vi "Dispatch Message.vi"(8 "error in (no error)":errorcluster, 10 "TcpPayload":T1, 11 "Remote Messaging Module in":refnum<class "Remote Messaging Module.lvclass">) -> (0 "error out":errorcluster, 3 "Remote Messaging Module out":refnum<class "Remote Messaging Module.lvclass">)   [LabVIEW 2020, in "Volatus.lvlib" / "Remote Messaging Module.lvclass"]
uses:
  Remote Messaging Module.lvclass
  C:/dev/lv20CE/relink/lv-volatus/Volatus/Module/Module.lvclass
  lv-vecto/Vecto/proto/TcpPayload/Data.ctl
  Module/Module.lvclass/Module.ctl
  Module Identity/Module Identity.lvclass/Module Identity.ctl
  MessageQ/MessageQ.lvclass/MessageQ.ctl
  Event Level.ctl
  Remote Messaging Module.lvclass/Remote Messaging Module.ctl
  Module Identity/Module Identity.lvclass
  C:/dev/lv20CE/relink/lv-volatus/Volatus/Identity/Identity.lvclass
  Module/Module.lvclass
  MessageQ/MessageQ.lvclass
  VolatusAPI/VolatusAPI.lvclass
  Volatus.lvlib
  lv-vecto/Vecto/proto/TcpPayload/TcpPayload.lvlib
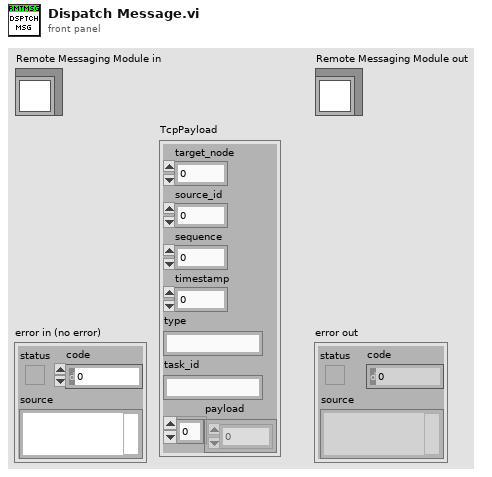
[diagram p1: front panel]
types:
  T1 = typedef "TcpPayload.lvlib/Data.ctl" = cluster{"target_node":u32, "source_id":u32, "sequence":u32, "timestamp":i64, "type":string, "task_id":string, "payload":u8[]}
  T2 = typedef "Volatus.lvlib/Event Level.ctl" = enum16{"Debug", "Info", "Warning", "Error"}
  T3 = typedef "Volatus.lvlib/Remote Messaging Module.lvclass/Type Handler.ctl" = cluster{"Msg ID":string, "MsgQ":refnum<class "MessageQ.lvclass">}
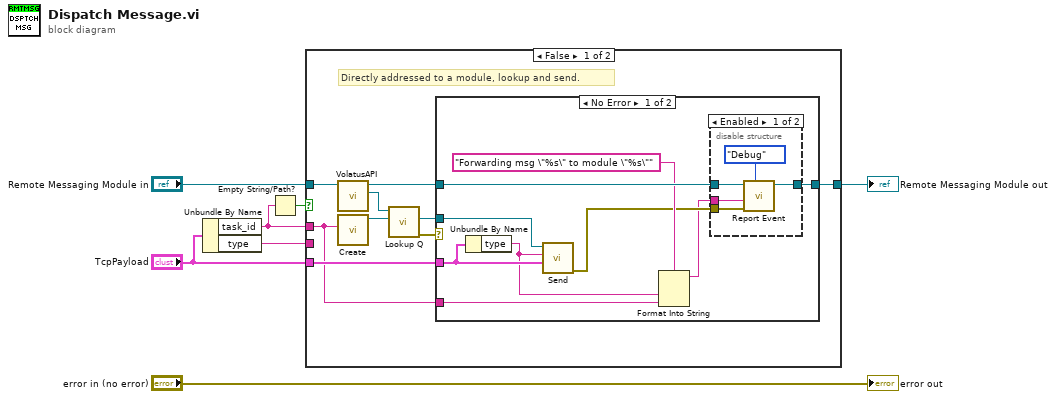
[diagram p0: block diagram]
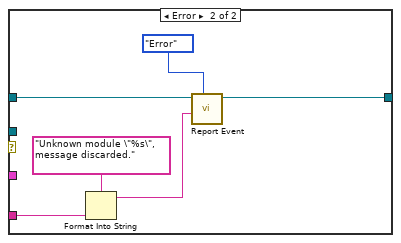
[diagram p3: hidden frame]
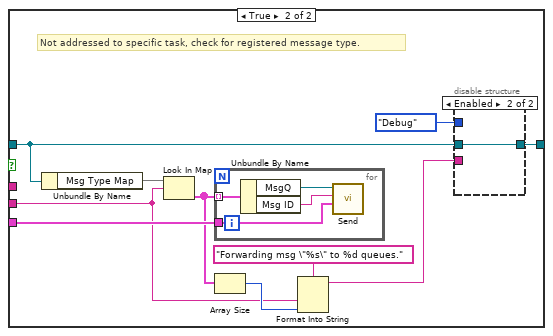
[diagram p4: hidden frame]
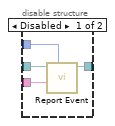
[diagram p5: hidden frame]
diagram:
  n1 = Unbundle By Name("TcpPayload") -> ("task_id"=w2:string, "type"=w4:string)
  n2 = Empty String/Path?(string/path=w2) -> (empty?=w5:bool)
  n3 = case shown="False" w5 {
    tunnel: "Remote Messaging Module in" -> [w16 w45]
    tunnel: w4 -> [_ w41]
    tunnel: "TcpPayload" -> [w11 w46]
    tunnel: w2 -> [w9 _]
    tunnel: [w8 w40] -> w1
    frame False {
      # "Directly addressed to a module, lookup and send."
      n4 = call "VolatusAPI.vi"("Module in"=w16) -> ("VolatusAPI"=w15:refnum<class "VolatusAPI.lvclass">, "Module out"=w10:refnum<class "Remote Messaging Module.lvclass">)  [unwired: 9 in]
      n5 = call "Create.vi"("ID"=w9) -> ("Module Identity out"=w14:refnum<class "Module Identity.lvclass">)  [unwired: 10 in]
      n6 = call "Lookup Q.vi"("Identity"=w14, "VolatusAPI in"=w15) -> ("error out"=w13:errorcluster, "MessageQ"=w12:refnum<class "MessageQ.lvclass">)  [unwired: 7 in, 1 out]
      n7 = case shown="No Error" w13 {
        tunnel: w12 -> [w25 _]
        tunnel: w11 -> [w24 _]
        tunnel: w10 -> [w23 w37]
        tunnel: w9 -> [w20 w34]
        tunnel: [w17 w32] -> w8
        frame No Error {
          n8 = Unbundle By Name(w24) -> ("type"=w21:string)
          n9 = call "Send.vi"("Data"=w24, "ID"=w21, "MessageQ in"=w25) -> ("error out"=w19:errorcluster)  [unwired: 7 in, 1 out]
          n10 = Format Into String(format string="Forwarding msg \"%s\" to module \"%s\"", w21, w20) -> (resulting string=w18:string)  [unwired: 2 in, 1 out]
          n11 = disable-structure shown="Enabled" {
            disable-tunnel: w23 -> [w30 w31]
            disable-tunnel: w19 -> [w29 _]
            disable-tunnel: w18 -> [w28 _]
            disable-tunnel: [w26 w31] -> w17
            frame Enabled {
              n12 = call "Report Event.vi"("Level (Info)"=Event_Level."Debug", "error in (no error)"=w29, "Message"=w28, "Module in"=w30) -> ("Module out"=w26:refnum<class "Remote Messaging Module.lvclass">)  [unwired: 6 in, 1 out]
            }
            frame Disabled {
            }
          }
        }
        frame Error {
          n13 = Format Into String(format string="Unknown module \"%s\", message discarded.", w34) -> (resulting string=w33:string)  [unwired: 2 in, 1 out]
          n14 = call "Report Event.vi"("Level (Info)"=Event_Level."Error", "Message"=w33, "Module in"=w37) -> ("Module out"=w32:refnum<class "Remote Messaging Module.lvclass">)  [unwired: 7 in, 1 out]
        }
      }
    }
    frame True {
      # "Not addressed to specific task, check for registered message type."
      n15 = Unbundle By Name(w45) -> ("Msg Type Map"=w47:map{string, T3[]})
      n16 = Look In Map(map=w47, key=w41) -> (value=w43:T3[])  [unwired: 1 in, 1 out]
      n17 = for {
        tunnel: w43 -> [w55] mode=indexing
        tunnel: w46 -> [w56]
        n18 = Unbundle By Name(w55) -> ("MsgQ"=w54:refnum<class "MessageQ.lvclass">, "Msg ID"=w53:string)
        n19 = call "Send.vi"("Data"=w56, "ID"=w53, "MessageQ in"=w54) -> ()  [unwired: 7 in, 2 out]
      }
      n20 = Array Size(array=w43) -> (size(s)=w42:i32)
      n21 = Format Into String(format string="Forwarding msg \"%s\" to %d queues.", w41, w42) -> (resulting string=w39:string)  [unwired: 2 in, 1 out]
      n22 = disable-structure shown="Enabled" {
        disable-tunnel: w45 -> [w51 w52]
        disable-tunnel: [w50 w52] -> w40
        disable-tunnel: w39 -> [w49 _]
        disable-tunnel: Event_Level."Debug" ("Level (Info)") -> [w48 _]
        frame Disabled {
          n23 = call "Report Event.vi"("Level (Info)"=w48, "Message"=w49, "Module in"=w51) -> ("Module out"=w50:refnum<class "Remote Messaging Module.lvclass">)  [unwired: 7 in, 1 out]
        }
        frame Enabled {
        }
      }
    }
  }
  "Remote Messaging Module out" <- w1
  "error out" <- "error in (no error)"
